vi "_MDPtr Pack Memory.vi"(6 "DT":T1, 7 "Copies Count(1)":i32=1, 9 "String Attribute":string, 10 "error in (no error)":errorcluster, 11 "String":string) -> (2 "error out":errorcluster, 3 "HexStrPtr":T2)   [LabVIEW 2017, in "MDPtr.lvlib"]
uses:
  MDPtr.lvlib
  MDPtr TypeDef/MDPtr.ctl
  <vilib>/Utility/Data Type/Type Definitions/Data Type.ctl
  _MDPtrMgr/MDPtrMgr.lvclass
  <vilib>/Utility/Data Type/NI_Data Type.lvlib
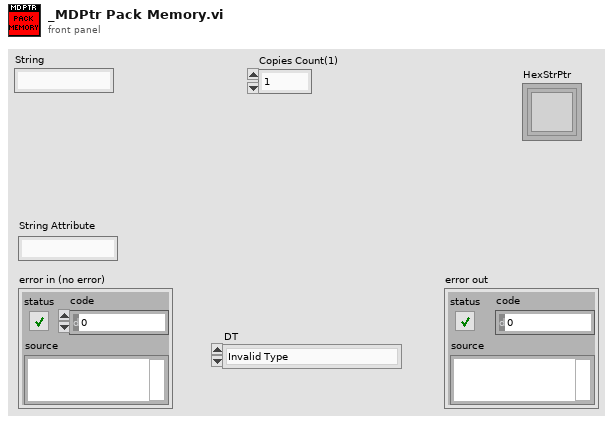
[diagram p1: front panel]
types:
  T1 = typedef "NI_Data Type.lvlib/Data Type.ctl" = enum8{"Invalid Type", "Void", "I8", "I16", "I32", "I64", "U8", "U16", "U32", "U64", "Single Float", "Double Float", "Extended Float", "Single Complex", "Double Complex", "Extended Complex", "Enum U8", "Enum U16", "Enum U32", "Enum U64", "Single Float With Unit", "Double Float With Unit", "Extended Float With Unit", "Single Complex with Unit", "Double Complex with Unit", "Extended Complex with Unit", "Boolean", "String", "Path", "Picture", "Tag", "Array", "Cluster", "Variant", "LV Variant", "Waveform", "Timestamp", "Digital Waveform", "Digital Data", "ExpressData", "Refnum", "External Data", "VI", "Poly VI", "LabVIEW Class Instance", "Fixed Point"}
  T2 = typedef "MDPtr.lvlib/MDPtr.ctl" = refnum<k1>
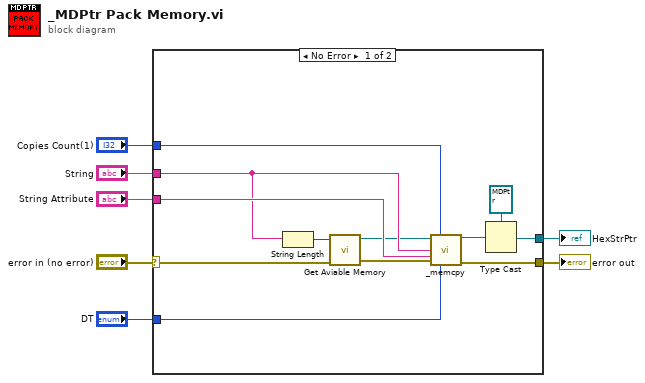
[diagram p0: block diagram]
diagram:
  n1 = case shown="No Error" "error in (no error)" {
    selector: "error in (no error)" -> [w10 w20]
    tunnel: [w19 w20] -> w6
    tunnel: "String" -> [w17 _]
    tunnel: [w13 _] -> w4
    tunnel: "Copies Count(1)" -> [w15 _]
    tunnel: "String Attribute" -> [w18 _]
    tunnel: "DT" -> [w16 _]
    frame No Error {
      n2 = String Length(string=w17) -> (length=w11:i32)
      n3 = call "Get Aviable Memory.vi"("error in (no error)"=w10, "DataLength"=w11) -> ("error out"=w8:errorcluster, "MDPtr DVR"=w9:refnum<data-value>)  [unwired: 8 in]
      n4 = call "_memcpy.vi"("MDPtr DVR"=w9, "Copy Count"=w15, "error in (no error)"=w8, "Memory"=w17, "String Attribute"=w18, "Data Type"=w16) -> ("MDPtr DVR(dup)"=w14:refnum<data-value>, "error out"=w19:errorcluster)  [unwired: 8 in]
      n5 = Type Cast(type=T2 refnum ("MDPtr"), x=w14) -> (*(type *) &x=w13:T2)
    }
    frame Error {
    }
  }
  "HexStrPtr" <- w4
  "error out" <- w6
